vi "getNewValueXML.vi"(8 "error in (no error)":errorcluster, 11 "RampEvent in":refnum<class "RampEvent.lvclass">) -> (0 "error out":errorcluster, 2 "newValueXML":refnum<class "xmlNode.lvclass">, 3 "RampEvent out":refnum<class "RampEvent.lvclass">)   [LabVIEW 2009, in "Tools.lvlib" / "Scripting.lvlib" / "RampEvent.lvclass"]
uses:
  RampEvent.lvclass
  xmlNode/xmlNode.lvclass
  ScriptEvent.lvclass
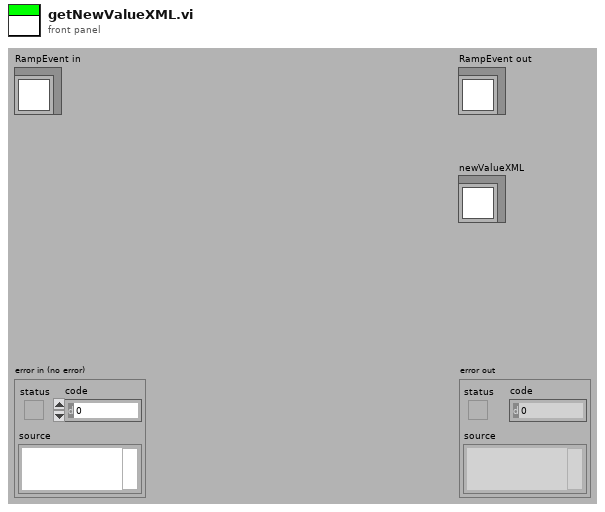
[diagram p1: front panel]
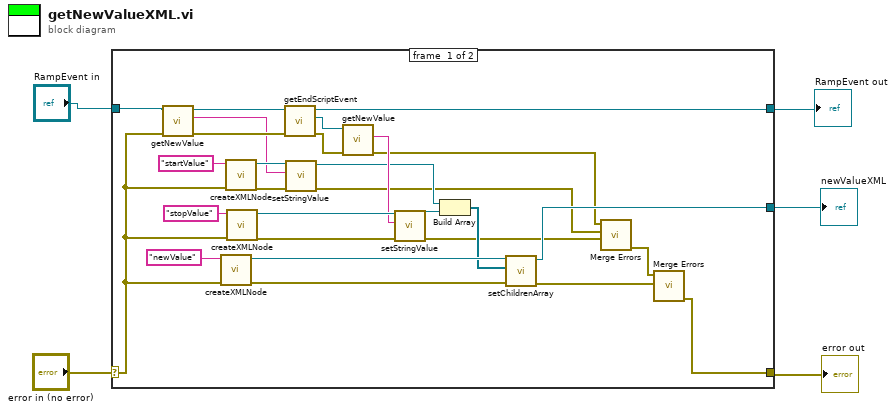
[diagram p0: block diagram]
diagram:
  n1 = case shown="No Error" "error in (no error)" {
    selector: "error in (no error)" -> [w26 w35]
    tunnel: [w6 w35] -> w3
    tunnel: [w32 w34] -> w4
    tunnel: "RampEvent in" -> [w31 w34]
    tunnel: [w15 _] -> w1
    frame #0 {
      n2 = call "getNewValue.vi"("error in (no error)"=w26, "ScriptEvent.lvclass in"=w31) -> ("error out"=w29:errorcluster, "newValue"=w23:string, "ScriptEvent.lvclass out"=w30:refnum<class "RampEvent.lvclass">)  [unwired: 7 in]
      n3 = call "createXMLNode.vi"("error in (no error)"=w26, "name"="newValue") -> ("error out"=w16:errorcluster, "xmlNode out"=w17:refnum<class "xmlNode.lvclass">)  [unwired: 8 in]
      n4 = call "createXMLNode.vi"("error in (no error)"=w26, "name"="startValue") -> ("error out"=w24:errorcluster, "xmlNode out"=w25:refnum<class "xmlNode.lvclass">)  [unwired: 8 in]
      n5 = call "createXMLNode.vi"("error in (no error)"=w26, "name"="stopValue") -> ("error out"=w21:errorcluster, "xmlNode out"=w22:refnum<class "xmlNode.lvclass">)  [unwired: 8 in]
      n6 = call "getEndScriptEvent.vi"("error in (no error)"=w29, "RampEvent.lvclass in"=w30) -> ("error out"=w20:errorcluster, "ScriptEvent.lvclass"=w19:refnum<class "ScriptEvent.lvclass">, "RampEvent.lvclass out"=w32:refnum<class "RampEvent.lvclass">)  [unwired: 7 in]
      n7 = call-dynamic "setStringValue.vi"("error in (no error)"=w24, "stringValue"=w23, "xmlNode.lvclass in"=w25) -> ("error out"=w10:errorcluster, "xmlNode.lvclass out"=w14:refnum<class "xmlNode.lvclass">)  [unwired: 7 in]
      n8 = call "getNewValue.vi"("error in (no error)"=w20, "ScriptEvent.lvclass in"=w19) -> ("error out"=w11:errorcluster, "newValue"=w18:string)  [unwired: 7 in, 1 out]
      n9 = call-dynamic "setStringValue.vi"("error in (no error)"=w21, "stringValue"=w18, "xmlNode.lvclass in"=w22) -> ("error out"=w9:errorcluster, "xmlNode.lvclass out"=w13:refnum<class "xmlNode.lvclass">)  [unwired: 7 in]
      n10 = Build Array(w14, w13) -> (w12:refnum<class "xmlNode.lvclass">[])
      n11 = call-dynamic "setChildrenArray.vi"("error in (no error)"=w16, "Children"=w12, "xmlNode.lvclass in"=w17) -> ("error out"=w7:errorcluster, "xmlNode.lvclass out"=w15:refnum<class "xmlNode.lvclass">)  [unwired: 7 in]
      n12 = call <vilib>:"Merge Errors.vi"("error in 3 (no error)"=w9, "error in 2 (no error)"=w10, "error in 1 (no error)"=w11) -> ("error out"=w8:errorcluster)  [unwired: 4 in]
      n13 = call <vilib>:"Merge Errors.vi"("error in 2 (no error)"=w7, "error in 1 (no error)"=w8) -> ("error out"=w6:errorcluster)  [unwired: 5 in]
    }
    frame #1 {
    }
  }
  "error out" <- w3
  "RampEvent out" <- w4
  "newValueXML" <- w1
